vi "SyncAudioTTL_SubVI_Backup.vi"(9 "Multiplier":dbl, 10 "Filter Type":u16(ring) items=["No filter", "4k high-pass", "4k-20k band-pass", "4k-50k band-pass"], 11 "Stimulus File":path) -> (0 "error out":errorcluster, 1 "digital waveform":digitalwaveform(waveform), 2 "task out 2":refnum<k21>, 3 "Refnum out":refnum<k21>, 4 "Stim File Length (s)":dbl, 5 "Array":waveform(dbl)[](array[waveform]))   [LabVIEW 2017]
uses:
  <vilib>/DAQmx/write.llb/DAQmx Write (Analog 1D Wfm NChan NSamp).vi
  <vilib>/DAQmx/write.llb/DAQmx Write (Digital Wfm 1Chan NSamp).vi
  <vilib>/DAQmx/miscellaneous.llb/DAQmx Fill In Error Info.vi
  <vilib>/Waveform/DWDTOps.llb/DWDT Uncompress Digital.vi
  <vilib>/DAQmx/configure/timing.llb/DAQmx Timing (Sample Clock).vi
  <vilib>/DAQmx/configure/trigger.llb/DAQmx Start Trigger (Digital Edge).vi
  <vilib>/Waveform/DWDTOps.llb/DWDT Analog to Digital.vi
  <vilib>/Waveform/WDTOps.llb/WDT Number of Waveform Samples DBL.vi
  <vilib>/DAQmx/create/channels.llb/DAQmx Create Channel (AO-Voltage-Basic).vi
  <vilib>/DAQmx/create/channels.llb/DAQmx Create Channel (DO-Digital Output).vi
  <resource>/objmgr/daqmx.rc
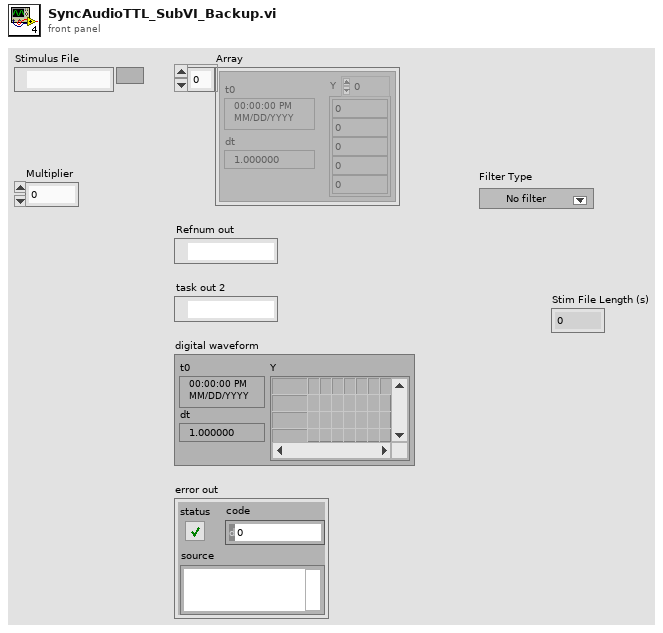
[diagram p1: front panel]
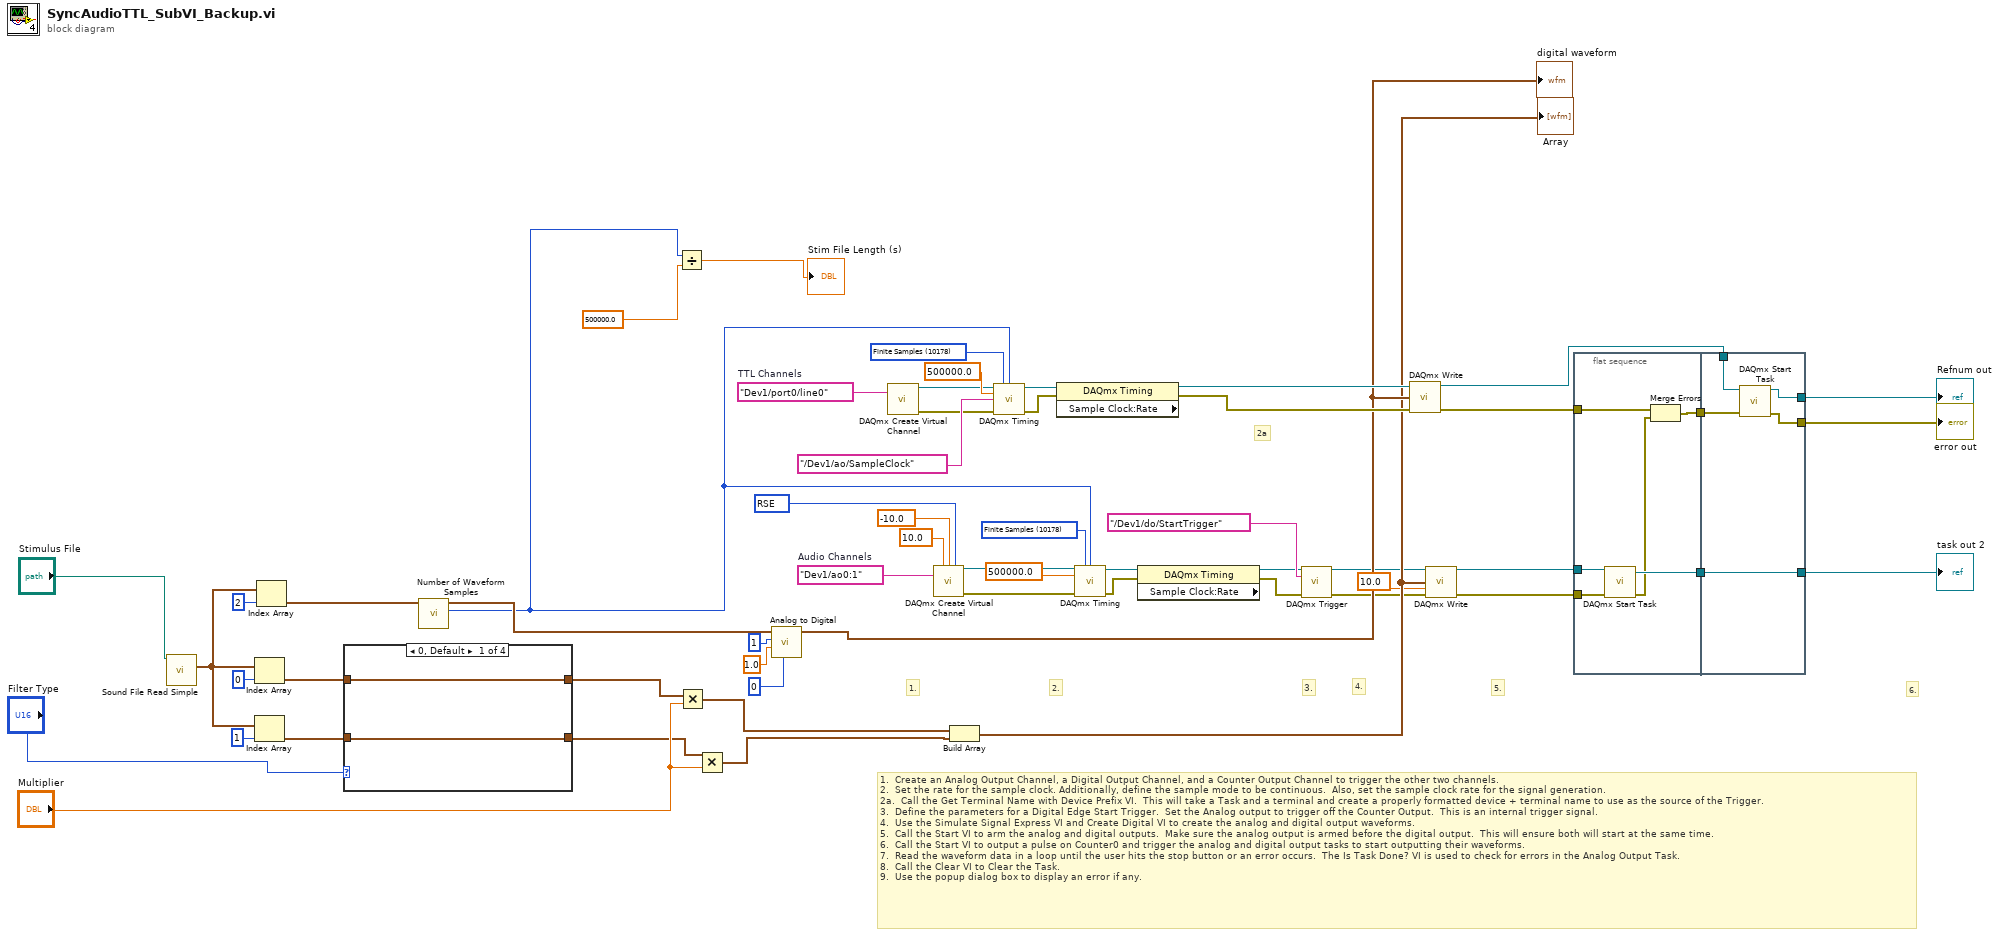
[diagram p0: block diagram]
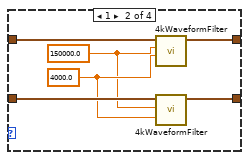
[diagram p2: hidden frame]
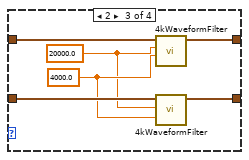
[diagram p3: hidden frame]
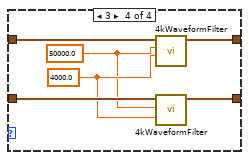
[diagram p4: hidden frame]
diagram:
  w56 = tag "Dev1/port0/line0"  # TTL Channels
  w55 = tag "Dev1/ao0:1"  # Audio Channels
  w52 = 10083 items=["Default"=-1, "RSE"=10083, "Differential"=10106, "Pseudodifferential"=12529] ("output terminal configuration")
  w10 = 10178 items=["Finite Samples"=10178, "Continuous Samples"=10123] ("sample mode")
  w5 = 10178 items=["Finite Samples"=10178, "Continuous Samples"=10123] ("sample mode")
  # "2a"
  # "6."
  # "3."
  # "4."
  # "5."
  # "1.  Create an Analog Output Channel, a Digital Output Channel, and a Counter Output Channel to trigger the other two channels.\n2.  Set the rate for the sample clock. Additionally, define the sample mode to be continuous.  Also, set the sample clock rate for the signal generation.\n2a.  Call the Get Terminal Name with Device Prefix VI.  This will take a Task and a terminal and create a properly formatted device + terminal name to use as the source of the Trigger.\n3.  Define the parameters for a Digital Edge Start Trigger.  Set the Analog output to trigger off the Counter Output.  This is an internal trigger signal.\n4.  Use the Simulate Signal Express VI and Create Digital VI to create the analog and digital output waveforms.\n5.  Call the Start VI to arm the analog and digital outputs.  Make sure the analog output is armed before the digital output.  This will ensure both will start at the same time.\n6.  Call the Start VI to output a pulse on Counter0 and trigger the analog and digital output tasks to start outputting their waveforms.\n7.  Read the waveform data in a loop until the user hits the stop button or an error occurs.  The Is Task Done? VI is used to check for errors in the Analog Output Task.\n8.  Call the Clear VI to Clear the Task.\n9.  Use the popup dialog box to display an error if any."
  # "2."
  # "1."
  n1 = call <vilib>:"Sound File Read Simple.vi"("path"="Stimulus File") -> ("data"=w32:waveform(dbl)[])  [unwired: 7 in, 3 out]
  n2 = Index Array(array=w32, index=0) -> (element=w36:waveform(dbl))
  n3 = Index Array(array=w32, index=1) -> (element=w40:waveform(dbl))
  n4 = Index Array(array=w32, index=2) -> (element=w50:waveform(dbl))
  n5 = case shown="0, Default" "Filter Type" {
    tunnel: w36 -> [w60 w66 w72 w78]
    tunnel: [w60 w65 w71 w77] -> w41
    tunnel: [w59 w64 w70 w76] -> w43
    tunnel: w40 -> [w59 w63 w69 w75]
    frame 0, Default {
    }
    frame 1 {
      w61 = 150000.0
      w62 = 4000.0
      n6 = call "4kWaveformFilter.vi"("Low cutoff"=w62, "High cutoff"=w61, "data"=w66) -> ("Waveform"=w65:waveform(dbl))  [unwired: 8 in]
      n7 = call "4kWaveformFilter.vi"("Low cutoff"=w62, "High cutoff"=w61, "data"=w63) -> ("Waveform"=w64:waveform(dbl))  [unwired: 8 in]
    }
    frame 2 {
      w67 = 20000.0
      w68 = 4000.0
      n8 = call "4kWaveformFilter.vi"("Low cutoff"=w68, "High cutoff"=w67, "data"=w72) -> ("Waveform"=w71:waveform(dbl))  [unwired: 8 in]
      n9 = call "4kWaveformFilter.vi"("Low cutoff"=w68, "High cutoff"=w67, "data"=w69) -> ("Waveform"=w70:waveform(dbl))  [unwired: 8 in]
    }
    frame 3 {
      w73 = 50000.0
      w74 = 4000.0
      n10 = call "4kWaveformFilter.vi"("Low cutoff"=w74, "High cutoff"=w73, "data"=w78) -> ("Waveform"=w77:waveform(dbl))  [unwired: 8 in]
      n11 = call "4kWaveformFilter.vi"("Low cutoff"=w74, "High cutoff"=w73, "data"=w75) -> ("Waveform"=w76:waveform(dbl))  [unwired: 8 in]
    }
  }
  n12 = call-poly <vilib>:"Number of Waveform Samples.vi"("waveform in"=w50) -> ("number of samples"=w4:i32, "waveform out"=w51:waveform(dbl))  [unwired: 8 in, 1 out]
  n13 = Divide(x=w4, y=500000.0) -> (x/y=→"Stim File Length (s)":dbl)
  n14 = Multiply(x=w41, y="Multiplier") -> (x*y=w42:waveform(dbl))
  n15 = Multiply(x=w43, y="Multiplier") -> (x*y=w44:waveform(dbl))
  n16 = call-poly <vilib>:"Analog to Digital.vi"("data format (offset binary)"=0, "full-scale range (pk-pk)"=1.0, "resolution (16 bit)"=1, "analog waveform"=w51) -> ("digital waveform"=w38:digitalwaveform)  [unwired: 4 in, 3 out]
  "digital waveform" <- w38
  n17 = call-poly <vilib>:"DAQmx Create Virtual Channel.vi"("lines"=w56) -> ("task out"=w7:refnum<k21>, "error out"=w6:errorcluster)  [unwired: 6 in, 7 out]
  n18 = call-poly <vilib>:"DAQmx Create Virtual Channel.vi"("maximum value"=10.0, "minimum value"=-10.0, "output terminal configuration"=w52, "physical channels"=w55) -> ("task out"=w11:refnum<k21>, "error out"=w12:errorcluster)  [unwired: 5 in, 5 out]
  n19 = Build Array(w42, w44) -> (w37:waveform(dbl)[])
  "Array" <- w37
  n20 = call-poly <vilib>:"DAQmx Timing.vi"("task/channels in"=w7, "sample mode"=w5, "samples per channel"=w4, "rate"=500000.0 ("Rate"), "source"=tag "/Dev1/ao/SampleClock", "error in"=w6) -> ("task out"=w25:refnum<k21>, "error out"=w28:errorcluster)  [unwired: 1 in, 7 out]
  n21 = property class="DAQmx Timing" props=["Sample Clock:Rate"](reference=w25, error in=w28) -> (reference out=w53:refnum<k21>, error out=w54:errorcluster)  [unwired: 1 out]
  n22 = call-poly <vilib>:"DAQmx Timing.vi"("task/channels in"=w11, "sample mode"=w10, "samples per channel"=w4, "rate"=500000.0, "error in"=w12) -> ("task out"=w22:refnum<k21>, "error out"=w23:errorcluster)  [unwired: 2 in, 7 out]
  n23 = property class="DAQmx Timing" props=["Sample Clock:Rate"](reference=w22, error in=w23) -> (reference out=w21:refnum<k21>, error out=w24:errorcluster)  [unwired: 1 out]
  n24 = call-poly <vilib>:"DAQmx Trigger.vi"("task/channels in"=w21, "source"=tag "/Dev1/do/StartTrigger", "error in"=w24) -> ("task out"=w19:refnum<k21>, "error out"=w18:errorcluster)  [unwired: 2 in, 9 out]
  n25 = call-poly <vilib>:"DAQmx Write.vi"("task/channels in"=w53, "data"=w38, "error in"=w54) -> ("task out"=w47:refnum<k21>, "error out"=w27:errorcluster)  [unwired: 2 in, 9 out]
  n26 = call-poly <vilib>:"DAQmx Write.vi"("task/channels in"=w19, "data"=w37, "timeout"=10.0 ("Wirite Timeout"), "error in"=w18) -> ("task out"=w16:refnum<k21>, "error out"=w17:errorcluster)  [unwired: 1 in, 9 out]
  n27 = flat-sequence {
    tunnel: w16 -> [w83]
    tunnel: w17 -> [w82]
    tunnel: w27 -> [w79]
    tunnel: [w84] -> w58
    tunnel: [w80] -> w57
    tunnel: [w89] -> w13
    tunnel: w58 -> [w89]
    tunnel: w57 -> [w87]
    tunnel: w47 -> [w88]
    tunnel: [w86] -> w48
    tunnel: [w85] -> w49
    frame #0 {
      n28 = call <vilib>:"DAQmx Start Task.vi"("task/channels in"=w83, "error in"=w82) -> ("task out"=w84:refnum<k21>, "error out"=w81:errorcluster)  [unwired: 12 out]
      n29 = Merge Errors(w79, w81) -> (w80:errorcluster)
    }
    frame #1 {
      n30 = call <vilib>:"DAQmx Start Task.vi"("task/channels in"=w88, "error in"=w87) -> ("task out"=w86:refnum<k21>, "error out"=w85:errorcluster)  [unwired: 12 out]
    }
  }
  "error out" <- w49
  "Refnum out" <- w48
  "task out 2" <- w13
